vi "Process Line Items WIP.vi"(8 "error in (no error)":errorcluster, 11 "Provisional Line Items Corrected":T1[](array[typedef]) {"PriceIncDiscount (£)" format="%.2g"; "Discount(£)" format="%.2g"}) -> (0 "error out":errorcluster, 1 "NumberOfItems 2":i32, 2 "Item.TotalDiscount 2":dbl[](array[numeric]), 3 "Item.TotalPriceIncludingDiscount 2":dbl[](array[numeric]))   [LabVIEW 2018, in "Main.lvlib"]
uses:
  Main.lvlib
  receipt parsing/ReceiptItemInfo.ctl
  receipt parsing/Receipt Parsing.lvlib
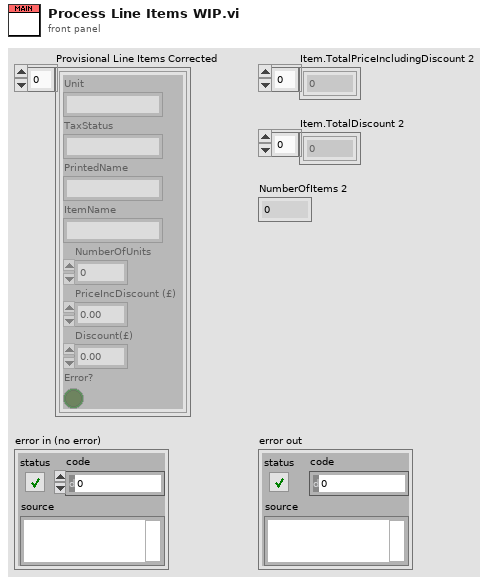
[diagram p1: front panel]
types:
  T1 = typedef "Receipt Parsing.lvlib/ReceiptItemInfo.ctl" = cluster{"Unit":string, "TaxStatus":string, "PrintedName":string, "ItemName":string, "NumberOfUnits":dbl, "PriceIncDiscount (£)":dbl, "Discount(£)":dbl, "Error?":bool}
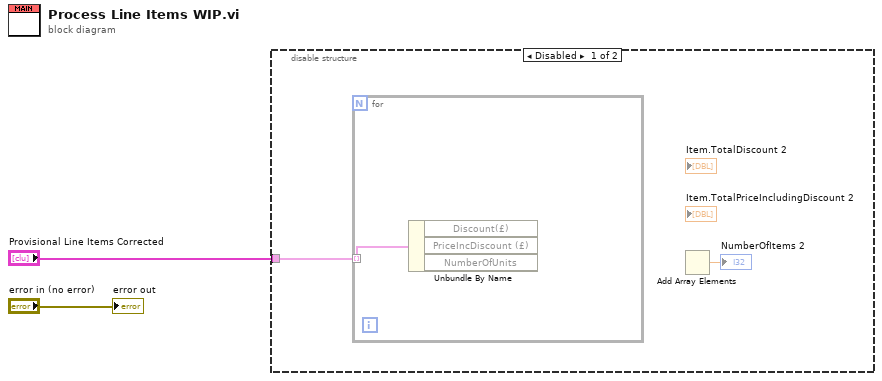
[diagram p0: block diagram]
diagram:
  n1 = disable-structure shown="Disabled" {
    disable-tunnel: "Provisional Line Items Corrected" -> [w3 _]
    frame Disabled {
      n2 = for {
        tunnel: w3 -> [w5] mode=indexing
        n3 = Unbundle By Name(w5) -> ()  [unwired: 3 out]
      }
      n4 = Add Array Elements() -> (sum=→"NumberOfItems 2":dbl)  [unwired: 1 in]
    }
    frame Enabled {
    }
  }
  "error out" <- "error in (no error)"
